vi "Route calulation.vi"(9 "Robot location":dbl[](array[numeric]), 10 "Target Location":dbl[](array[numeric]), 11 "Display Map":dbl[][](array[numeric])) -> (2 "Route map":dbl[][](array[numeric]), 3 "New display map":dbl[][](array[numeric]))   [LabVIEW 2015]
uses:
  <vilib>/robotics/Navigation/shared/WorldMap/OccupancyGridWorldMap/NI_Robotics_OccupancyGridWorldMap.lvclass
  <vilib>/robotics/Navigation/NI_Robotics_Navigation .lvlib
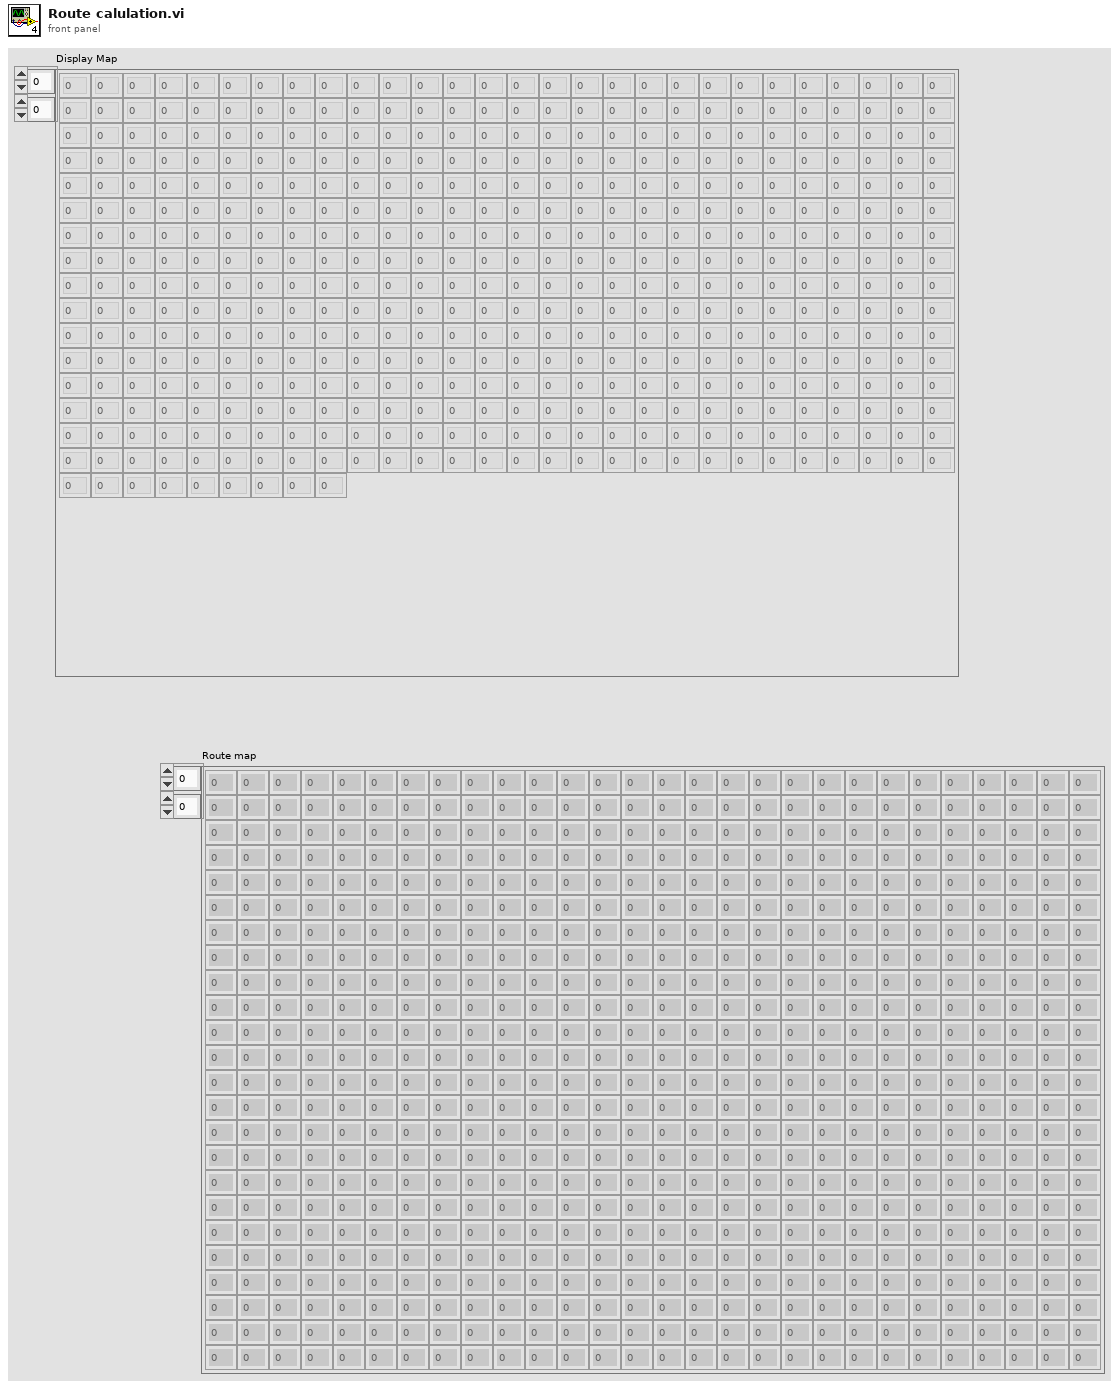
[diagram p1: front panel]
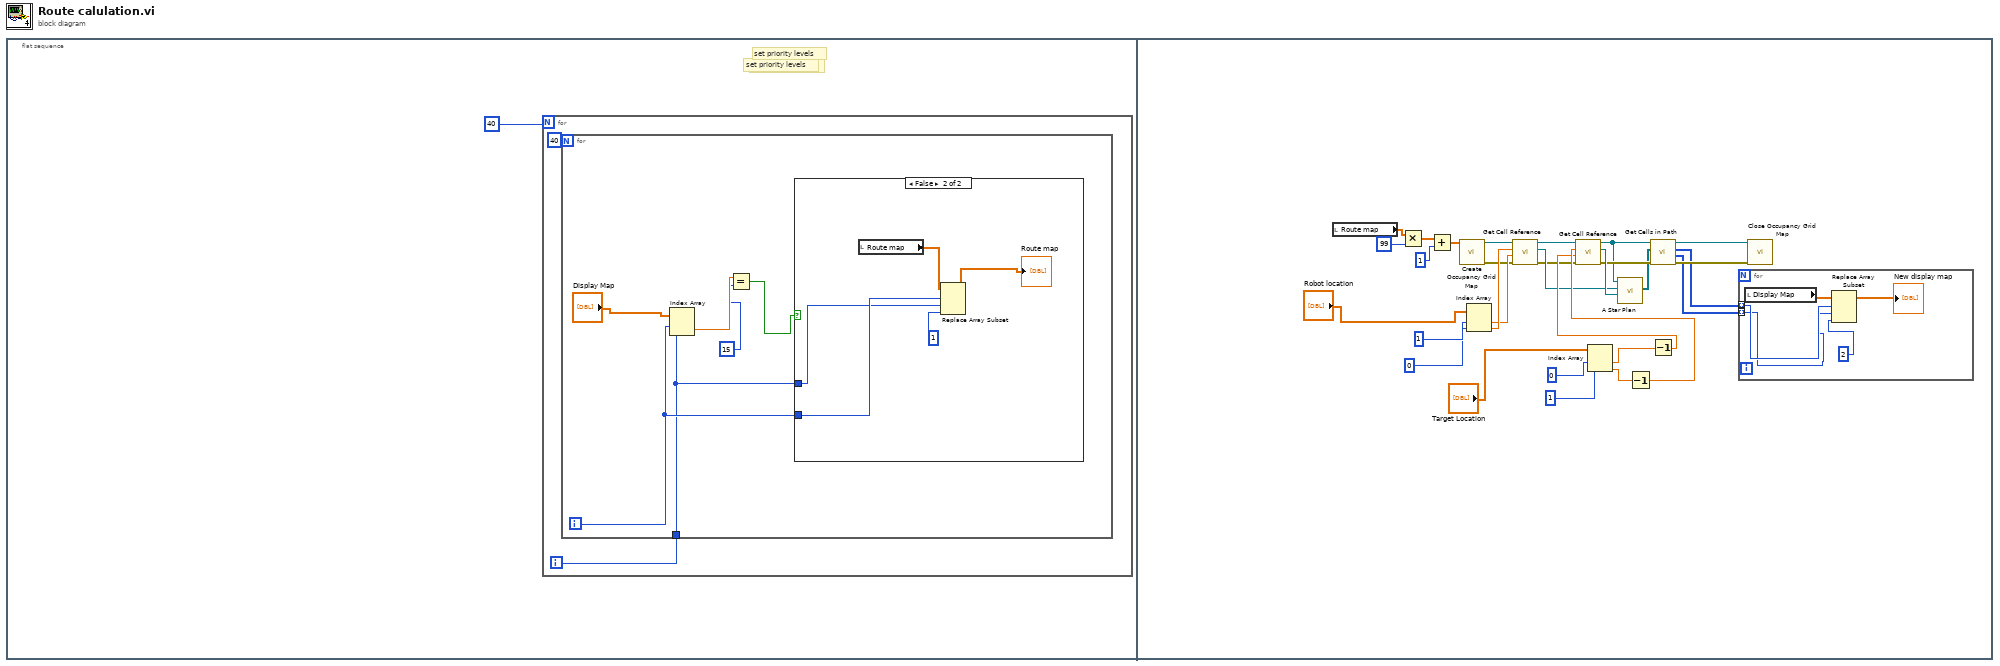
[diagram p0: block diagram]
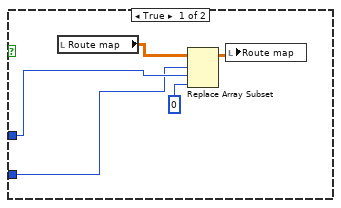
[diagram p2: hidden frame]
diagram:
  n1 = flat-sequence {
    frame #0 {
      # "set priority levels"
      # "set priority levels"
      # "set priority levels"
      n2 = for {
        N: 40 -> [_]
        i -> [w2]
        n3 = for {
          N: 40 -> [_]
          tunnel: w2 -> [w8]
          i -> [w9]
          n4 = Index Array(array="Display Map", index (row)=w9, index (col)=w8) -> (element=w6:dbl)
          n5 = Equal?(x=w6, y=15) -> (x = y?=w7:bool)
          n6 = case shown="False" w7 {
            tunnel: w9 -> [w10 w17]
            tunnel: w8 -> [w11 w16]
            frame True {
              n7 = local read "Route map"() -> (w13:dbl[][])
              n8 = Replace Array Subset(array=w13, new element=0, index (row)=w10, index (col)=w11) -> (w14:dbl[][])
              n9 = local write "Route map"(w14) -> ()
            }
            frame False {
              n10 = local read "Route map"() -> (w18:dbl[][])
              n11 = Replace Array Subset(array=w18, new element=1, index (row)=w17, index (col)=w16) -> (→"Route map":dbl[][])
            }
          }
        }
      }
    }
    frame #1 {
      n12 = local read "Route map"() -> (w39:dbl[][])
      n13 = Multiply(x=w39, y=99) -> (x*y=w28:dbl[][])
      n14 = Add(x=w28, y=1) -> (x+y=w30:dbl[][])
      n15 = call <vilib>:"Create Occupancy Grid Map.vi"("occupancy grid"=w30) -> ("error out"=w31:errorcluster, "map reference out"=w35:refnum<data-value>)  [unwired: 9 in]
      n16 = Index Array(array="Robot location", index #1=0, index #2=1) -> (element #1=w48:dbl, element #2=w49:dbl)
      n17 = call <vilib>:"Get Cell Reference.vi"("error in (no error)"=w31, "y"=w48, "x"=w49, "map reference in"=w35) -> ("error out"=w32:errorcluster, "cell reference"=w34:refnum<data-value>, "map reference out"=w22:refnum<data-value>)  [unwired: 4 in, 1 out]
      n18 = Index Array(array="Target Location", index #1=0, index #2=1) -> (element #1=w44:dbl, element #2=w45:dbl)
      n19 = Decrement(x=w45) -> (x-1=w47:dbl)
      n20 = Decrement(x=w44) -> (x-1=w46:dbl)
      n21 = call <vilib>:"Get Cell Reference.vi"("error in (no error)"=w32, "y"=w46, "x"=w47, "map reference in"=w22) -> ("error out"=w33:errorcluster, "cell reference"=w36:refnum<data-value>, "map reference out"=w24:refnum<data-value>)  [unwired: 4 in, 1 out]
      n22 = call <vilib>:"A Star Plan.vi"("goal reference"=w36, "start reference"=w34, "map reference in"=w24) -> ("path references"=w23:refnum<data-value>[])  [unwired: 5 in, 3 out]
      n23 = call <vilib>:"Get Cells in Path.vi"("error in (no error)"=w33, "path references"=w23, "map reference in"=w24) -> ("error out"=w38:errorcluster, "y coordinates"=w25:i32[], "x coordinates"=w26:i32[], "map reference out"=w37:refnum<data-value>)  [unwired: 5 in]
      n24 = for {
        tunnel: w25 -> [w53] mode=indexing
        tunnel: w26 -> [w54] mode=indexing
        n25 = local read "Display Map"() -> (w51:dbl[][])
        n26 = Replace Array Subset(array=w51, new element=2, index (row)=w54, index (col)=w53) -> (→"New display map":dbl[][])
      }
      n27 = call <vilib>:"Close Occupancy Grid Map.vi"("error in (no error)"=w38, "map reference in"=w37) -> ()  [unwired: 9 in, 1 out]
    }
  }
